vi "add_JointPositions.vi"(3 "Names":string[](array[string]), 4 "Angles":dbl[](array[numeric]), 5 "msg in":string) -> (2 "msg out":string)   [LabVIEW 2013]
uses:
  Primitives/subs/float64Array.vi
  Primitives/subs/stringArray.vi
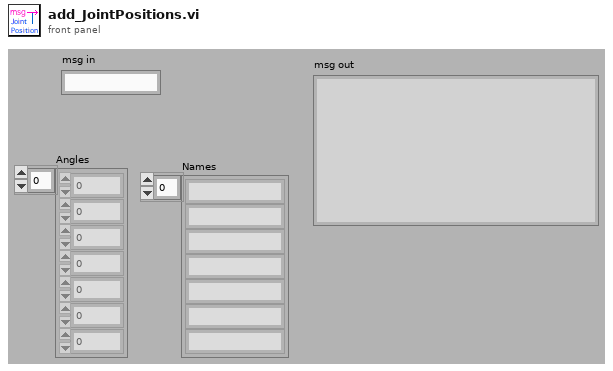
[diagram p1: front panel]
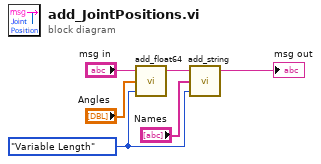
[diagram p0: block diagram]
diagram:
  w3 = enum16{"Fixed Length", "Variable Length"}."Variable Length" ("Array Type")
  n1 = call-poly "add_float64.vi"("Array Type"=w3, "Array"="Angles", "msg in"="msg in") -> ("msg out"=w5:string)  [unwired: 2 in]
  n2 = call-poly "add_string.vi"("Array Type"=w3, "Array"="Names", "msg in"=w5) -> ("msg out"=→"msg out":string)  [unwired: 2 in]
